vi "CheckCore.vi"(8 "error in (no error)":errorcluster, 9 "# of Refs":i32, 10 "References":refnum<vi>[](array[refnum]), 11 "Invoke in":refnum<class "Invoke.lvclass">) -> (0 "error out":errorcluster, 1 "Reject?":bool, 2 "dup References":refnum<vi>[](array[refnum]), 3 "Invoke out":refnum<class "Invoke.lvclass">)   [LabVIEW 2014, in "lvbuildsecurity.lvlib" / "Invoke.lvclass"]
uses:
  Invoke.lvclass
  Blacklist.lvclass/Blacklist.ctl
  ReadVIRefnum.vi
  ReadCLI.vi
  ReadItems.vi
  <vilib>/Wiresmith Technology/LabVIEW CLI/CLI Class/CLI.lvclass
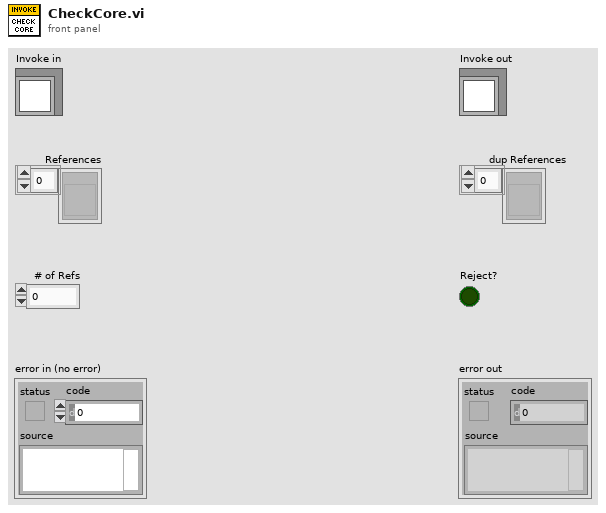
[diagram p1: front panel]
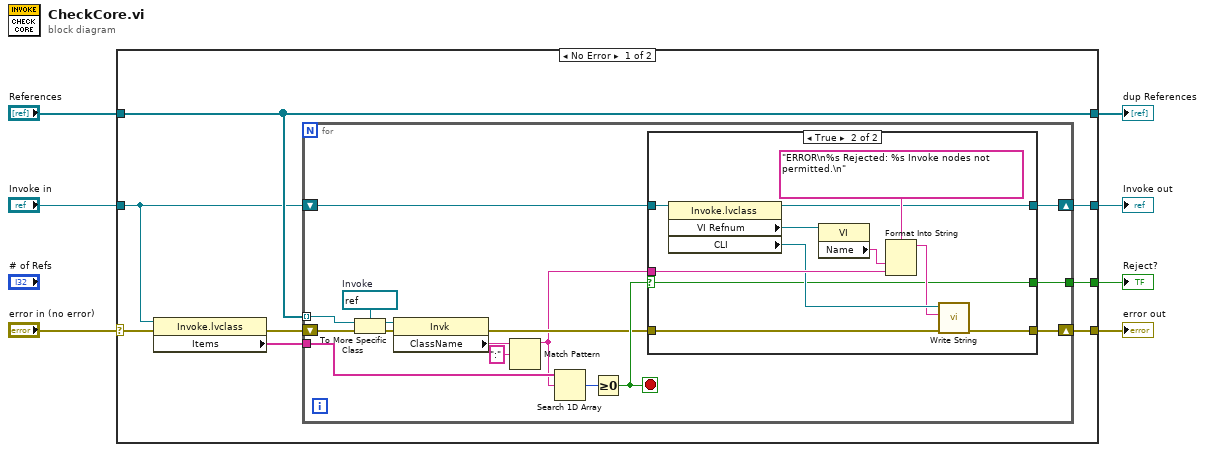
[diagram p0: block diagram]
diagram:
  n1 = case shown="No Error" "error in (no error)" {
    selector: "error in (no error)" -> [w13 w48]
    tunnel: [w15 w48] -> w6
    tunnel: "References" -> [w14 w46]
    tunnel: "Invoke in" -> [w9 w47]
    tunnel: [w8 w47] -> w3
    tunnel: [w14 w46] -> w2
    tunnel: [w10 _] -> w1
    frame No Error {
      n2 = property class="Invoke.lvclass"(reference=w9, error in=w13) -> (error out=w12:errorcluster, "Items"=w11:string[])  [unwired: 1 out]
      n3 = for {
        tunnel: w14 -> [w30] mode=indexing
        shift-right: [w19] -> w15
        shift-left: w12 -> [w31]
        tunnel: w11 -> [w26]
        tunnel: [w17] -> w10
        shift-right: [w21] -> w8
        shift-left: w9 -> [w22]
        stop <- w20 stop-if-true
        w29 = refnum<vi> refnum  # Invoke
        n4 = To More Specific Class(target class=w29, reference=w30, error in=w31) -> (specific class reference=w27:refnum<vi>, error out=w28:errorcluster)
        n5 = property class="Invk"(reference=w27, error in=w28) -> (error out=w18:errorcluster, "ClassName"=w23:string)  [unwired: 1 out]
        n6 = Match Pattern(string=w23, regular expression=":") -> (before substring=w16:string)  [unwired: 1 in, 3 out]
        n7 = Search 1D Array(1D array=w26, element=w16) -> (index of element=w25:i32)  [unwired: 1 in]
        n8 = Greater Or Equal To 0?(x=w25) -> (x >= 0?=w20:bool)
        n9 = case shown="True" w20 {
          selector: w20 -> [w32 w35]
          tunnel: w22 -> [w34 w45]
          tunnel: [w34 w38] -> w21
          tunnel: w16 -> [_ w41]
          tunnel: w18 -> [w33 w37]
          tunnel: [w33 w36] -> w19
          tunnel: [w32 w35] -> w17
          frame False {
          }
          frame True {
            n10 = property class="Invoke.lvclass"(reference=w45) -> (reference out=w38:refnum<class "Invoke.lvclass">, "VI Refnum"=w43:refnum<vi>, "CLI"=w40:refnum<class "CLI.lvclass">)  [unwired: 1 in, 1 out]
            n11 = property class="VI"(reference=w43) -> ("Name"=w42:string)  [unwired: 1 in, 2 out]
            n12 = Format Into String(format string="ERROR\n%s Rejected: %s Invoke nodes not permitted.\n", w42, w41) -> (resulting string=w39:string)  [unwired: 2 in, 1 out]
            n13 = call <vilib>:"Write String.vi"("error in (no error)"=w37, "Text to Write"=w39, "CLI in"=w40) -> ("error out"=w36:errorcluster)  [unwired: 7 in, 1 out]
          }
        }
      }
    }
    frame Error {
    }
  }
  "error out" <- w6
  "Invoke out" <- w3
  "dup References" <- w2
  "Reject?" <- w1
